vi "Close.vi"(8 "error in (no error)":errorcluster, 11 "Data in":refnum<class "Multi_Bus.lvclass">) -> (0 "error out":errorcluster, 3 "Data out":refnum<class "Multi_Bus.lvclass">)   [LabVIEW 2021, in "Multi_Bus.lvclass"]
uses:
  Multi_Bus.lvclass
  <vilib>/TSA/Abstract Data Classes/Abs_Types/Type/Abs_Type.lvclass
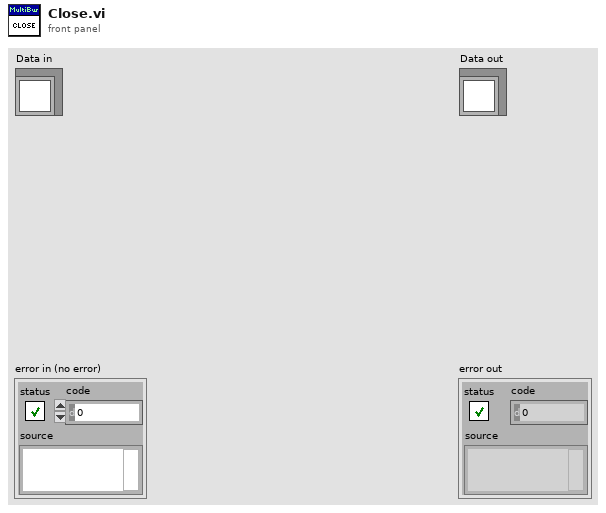
[diagram p1: front panel]
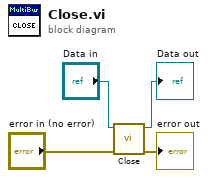
[diagram p0: block diagram]
diagram:
  n1 = call-parent "Close.vi"("error in (no error)"="error in (no error)", "Data in"="Data in") -> ("error out"=→"error out":errorcluster, "Data out"=→"Data out":refnum<class "Multi_Bus.lvclass">)  [unwired: 8 in]
